vi "Remove Duplicates 2D.vi"(2 "Which column/row":i32, 3 "By column/row":bool, 4 "Array in":i32[][](array[numeric])=[[1, 1, 2], [2, 3, 4], [2, 5, 5], [3, 5, 6], [3, 5, 8], [5, 7, 8], [5, 8, 15]]) -> (0 "Unique dimensions":i32, 1 "Array out":i32[][](array[numeric]))   [LabVIEW 2013]
doc: "The Remove Duplicates 2D VI removes rows or columns with a duplicate value in a sorted 2D array. First, you manually must sort each input array column and row in ascending or descending order to ensure the VI returns correct values. The VI searches in the row or column you specify, removing the entire row or column when the VI encounters a duplicate value. For example, if you specify the second column, the VI searches down that column and removes any row with a duplicate value in the second column. To specify search by row or column, use the By Column/Row control."
panel:
  # "Select Help»Show Context Help and move the cursor \nover the VI icon to display help for this VI."
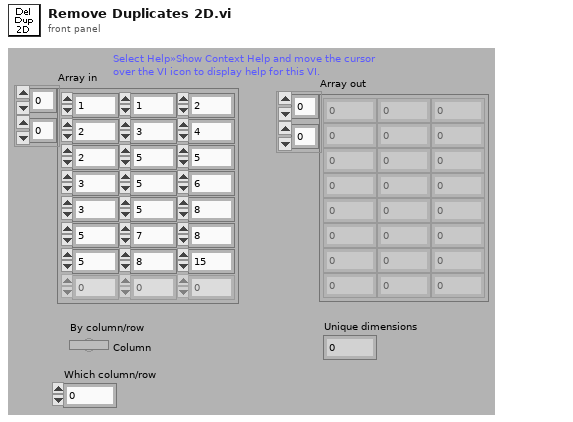
[diagram p1: front panel]
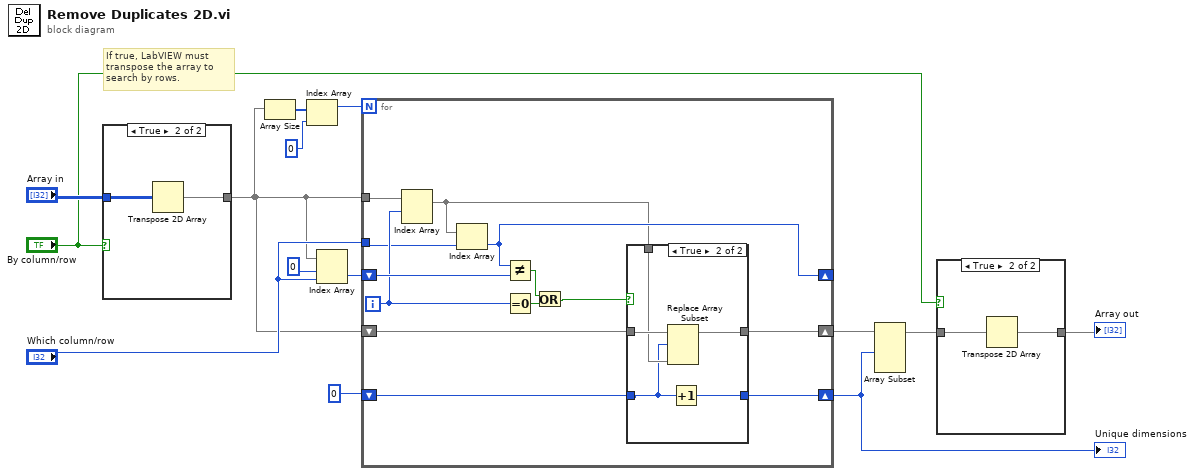
[diagram p0: block diagram]
diagram:
  # "If true, LabVIEW must transpose the array to search by rows."
  n1 = case shown="True" "By column/row" {
    tunnel: "Array in" -> [w15 w17]
    tunnel: [w15 w16] -> w4
    frame False {
    }
    frame True {
      n2 = Transpose 2D Array(2D array=w17) -> (transposed array=w16:i32[][])
    }
  }
  n3 = Array Size(array=w4) -> (size(s)=w8:i32[])
  n4 = Index Array "Index Array"(array=w8, index=0) -> (element=w6:i32)
  n5 = Index Array(array=w4, index (row)=0 ("index"), index (col)="Which column/row") -> (element=w14:i32)
  n6 = for {
    N: w6 -> [_]
    tunnel: w4 -> [w18]
    shift-right: [w21] -> _
    shift-left: w14 -> [w28]
    shift-right: [w26] -> w10
    shift-left: w4 -> [w27]
    shift-right: [w24] -> w9
    shift-left: 0 ("index") -> [w25]
    tunnel: "Which column/row" -> [w22]
    i -> [w23]
    n7 = Index Array "Index Array"(array=w18, index (row)=w23) -> (element=w19:i32[])  [unwired: 1 in]
    n8 = Index Array "Index Array"(array=w19, index=w22) -> (element=w21:i32)
    n9 = Not Equal?(x=w21, y=w28) -> (x != y?=w29:bool)
    n10 = Equal To 0?(x=w23) -> (x = 0?=w30:bool)
    n11 = Or(x=w29, y=w30) -> (x .or. y?=w20:bool)
    n12 = case shown="True" w20 {
      tunnel: w27 -> [w32 w37]
      tunnel: [w32 w33] -> w26
      tunnel: w19 -> [_ w36]
      tunnel: w25 -> [w31 w34]
      tunnel: [w31 w35] -> w24
      frame False {
      }
      frame True {
        n13 = Replace Array Subset "Replace Array Subset"(array=w37, new element=w36, index (row)=w34) -> (w33:i32[][])  [unwired: 1 in]
        n14 = Increment(x=w34) -> (x+1=w35:i32)
      }
    }
  }
  "Unique dimensions" <- w9
  n15 = Array Subset "Array Subset"(array=w10, length (row)=w9) -> (w3:i32[][])  [unwired: 3 in]
  n16 = case shown="True" "By column/row" {
    tunnel: w3 -> [w38 w40]
    tunnel: [w38 w39] -> w2
    frame False {
    }
    frame True {
      n17 = Transpose 2D Array(2D array=w40) -> (transposed array=w39:i32[][])
    }
  }
  "Array out" <- w2
